vi "Cluster_to_string_(SubVI).vi"(0 "input cluster 1":T1, 5 "input cluster 2":T1, 7 "input cluster 3":T1, 9 "input cluster 4":T1, 11 "error in":errorcluster) -> (8 "string of coefficients":string, 15 "error out":errorcluster)   [LabVIEW 2013]
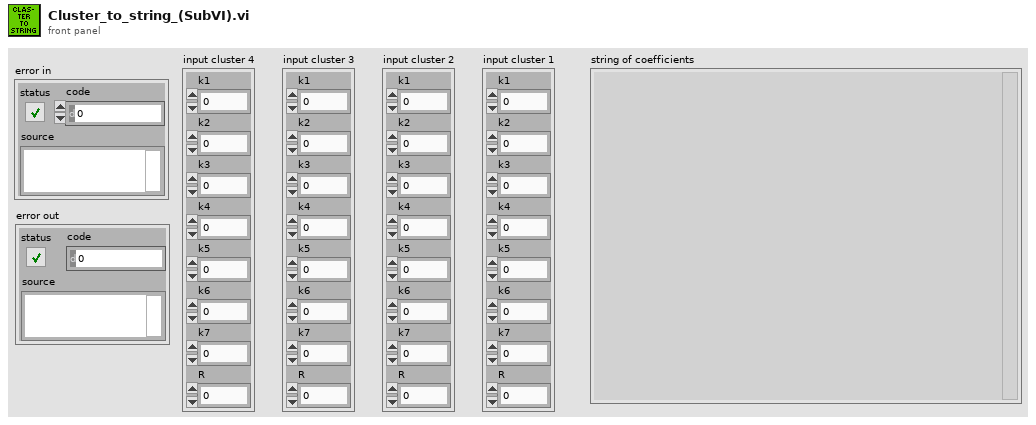
[diagram p1: front panel]
types:
  T1 = cluster{"k1":dbl, "k2":dbl, "k3":dbl, "k4":dbl, "k5":dbl, "k6":dbl, "k7":dbl, "R":dbl}
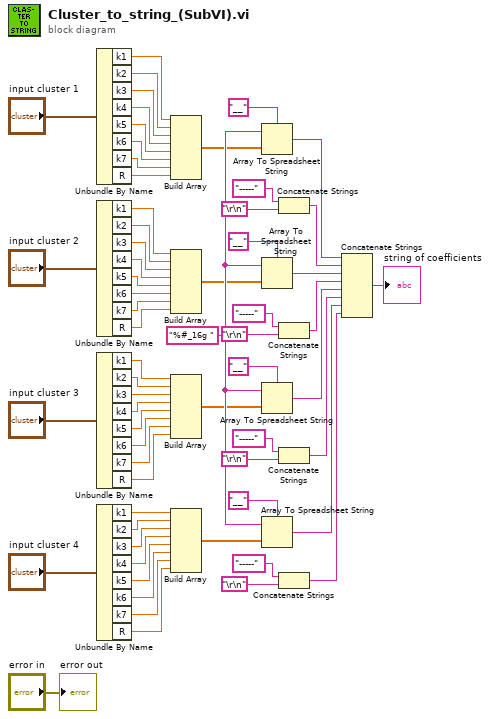
[diagram p0: block diagram]
diagram:
  w63 = "%#_16g " ("format string")
  n1 = Unbundle By Name("input cluster 1") -> ("k1"=w42:dbl, "k2"=w43:dbl, "k3"=w44:dbl, "k4"=w45:dbl, "k5"=w46:dbl, "k6"=w47:dbl, "k7"=w48:dbl, "R"=w49:dbl)
  n2 = Unbundle By Name("input cluster 2") -> ("k1"=w51:dbl, "k2"=w52:dbl, "k3"=w53:dbl, "k4"=w54:dbl, "k5"=w55:dbl, "k6"=w56:dbl, "k7"=w57:dbl, "R"=w58:dbl)
  n3 = Unbundle By Name("input cluster 3") -> ("k1"=w30:dbl, "k2"=w31:dbl, "k3"=w32:dbl, "k4"=w33:dbl, "k5"=w34:dbl, "k6"=w35:dbl, "k7"=w36:dbl, "R"=w37:dbl)
  n4 = Unbundle By Name("input cluster 4") -> ("k1"=w22:dbl, "k2"=w23:dbl, "k3"=w24:dbl, "k4"=w25:dbl, "k5"=w26:dbl, "k6"=w27:dbl, "k7"=w28:dbl, "R"=w29:dbl)
  n5 = Build Array(w42, w43, w44, w45, w46, w47, w48, w49) -> (w41:dbl[])
  n6 = Build Array(w51, w52, w53, w54, w55, w56, w57, w58) -> (w50:dbl[])
  n7 = Build Array(w30, w31, w32, w33, w34, w35, w36, w37) -> (w38:dbl[])
  n8 = Build Array(w22, w23, w24, w25, w26, w27, w28, w29) -> (w39:dbl[])
  n9 = Array To Spreadsheet String(delimiter (Tab)="__", array=w41, 3:w63) -> (spreadsheet string=w59:string)
  n10 = Array To Spreadsheet String(delimiter (Tab)="__", array=w50, 3:w63) -> (spreadsheet string=w60:string)
  n11 = Array To Spreadsheet String(delimiter (Tab)="__", array=w38, 3:w63) -> (spreadsheet string=w61:string)
  n12 = Array To Spreadsheet String(delimiter (Tab)="__", array=w39, 3:w63) -> (spreadsheet string=w62:string)
  n13 = Concatenate Strings("-----" ("string"), "\r\n") -> (w15:string)
  n14 = Concatenate Strings("-----" ("string"), "\r\n") -> (w13:string)
  n15 = Concatenate Strings("-----" ("string"), "\r\n") -> (w11:string)
  n16 = Concatenate Strings("-----" ("string"), "\r\n") -> (w1:string)
  n17 = Concatenate Strings(w59, w15, w60, w13, w61, w11, w62, w1) -> (→"string of coefficients":string)
  "error out" <- "error in"
